vi "PID2.vi"(8 "Boolean":bool, 11 "Numeric in":dbl) -> (3 "Numeric out":dbl)   [LabVIEW 2018]
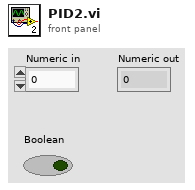
[diagram p1: front panel]
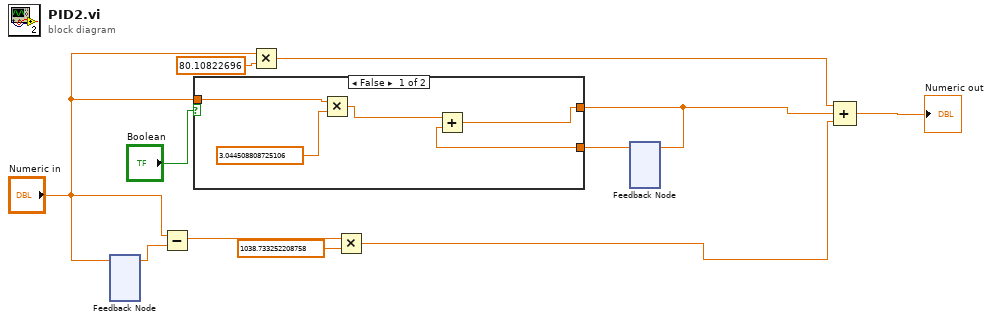
[diagram p0: block diagram]
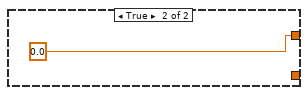
[diagram p2: hidden frame]
diagram:
  n1 = feedback #1() -> (w11:dbl)  [unwired: 1 in]
  n2 = feedback-in #1("Numeric in") -> ()
  n3 = Subtract(x="Numeric in", y=w11) -> (x-y=w7:dbl)
  n4 = Multiply(x="Numeric in", y=80.10822696) -> (x*y=w9:dbl)
  n5 = Multiply(x=w7, y=1038.733252208758) -> (x*y=w6:dbl)
  n6 = feedback #2() -> (w2:dbl)  [unwired: 1 in]
  n7 = case shown="False" "Boolean" {
    tunnel: "Numeric in" -> [w15 _]
    tunnel: [w13 0.0 ("x")] -> w1
    tunnel: w2 -> [w12 _]
    frame False {
      n8 = Multiply(x=w15, y=3.044508808725106 ("x")) -> (x*y=w14:dbl)
      n9 = Add(x=w14, y=w12) -> (x+y=w13:dbl)
    }
    frame True {
    }
  }
  n10 = feedback-in #2(w1) -> ()
  n11 = Compound Arithmetic op=ADD(w9, w1, w6) -> (→"Numeric out":dbl)
